vi "E517_InitialisationOfWaveScan.vi"(0 "amplitude":dbl, 5 "FastAxisStart":dbl, 7 "Fast Axis":string="1", 8 "Slow Axis Steps":dbl, 11 "error in":errorcluster, 12 "FastAxisStepsize":dbl, 13 "kineticexposure":dbl) -> (4 "scan time for 1 line/sec":dbl=200.0 format="%.3g", 6 "scan time for 1 area/sec 2":dbl=200.0 format="%.3g", 15 "error out 2":errorcluster)   [LabVIEW 2011]
doc: "This VI initializes and configures the E-710 to perform a XY scan."
uses:
  Utilities/controls/ctlSeqFNs_PI_SysNr.ctl
  Variables/GlobalSetNumberOfDigits_PhysikalInstruments.vi
panel:
  # "E-710 Wavescan Initialization"
  # "This VI initializes and configures the E-710 to perform a XY raster scan. Scan motion in X axis can be uni-\nor bidirectional. Triggerline 1 fires on waveform start."
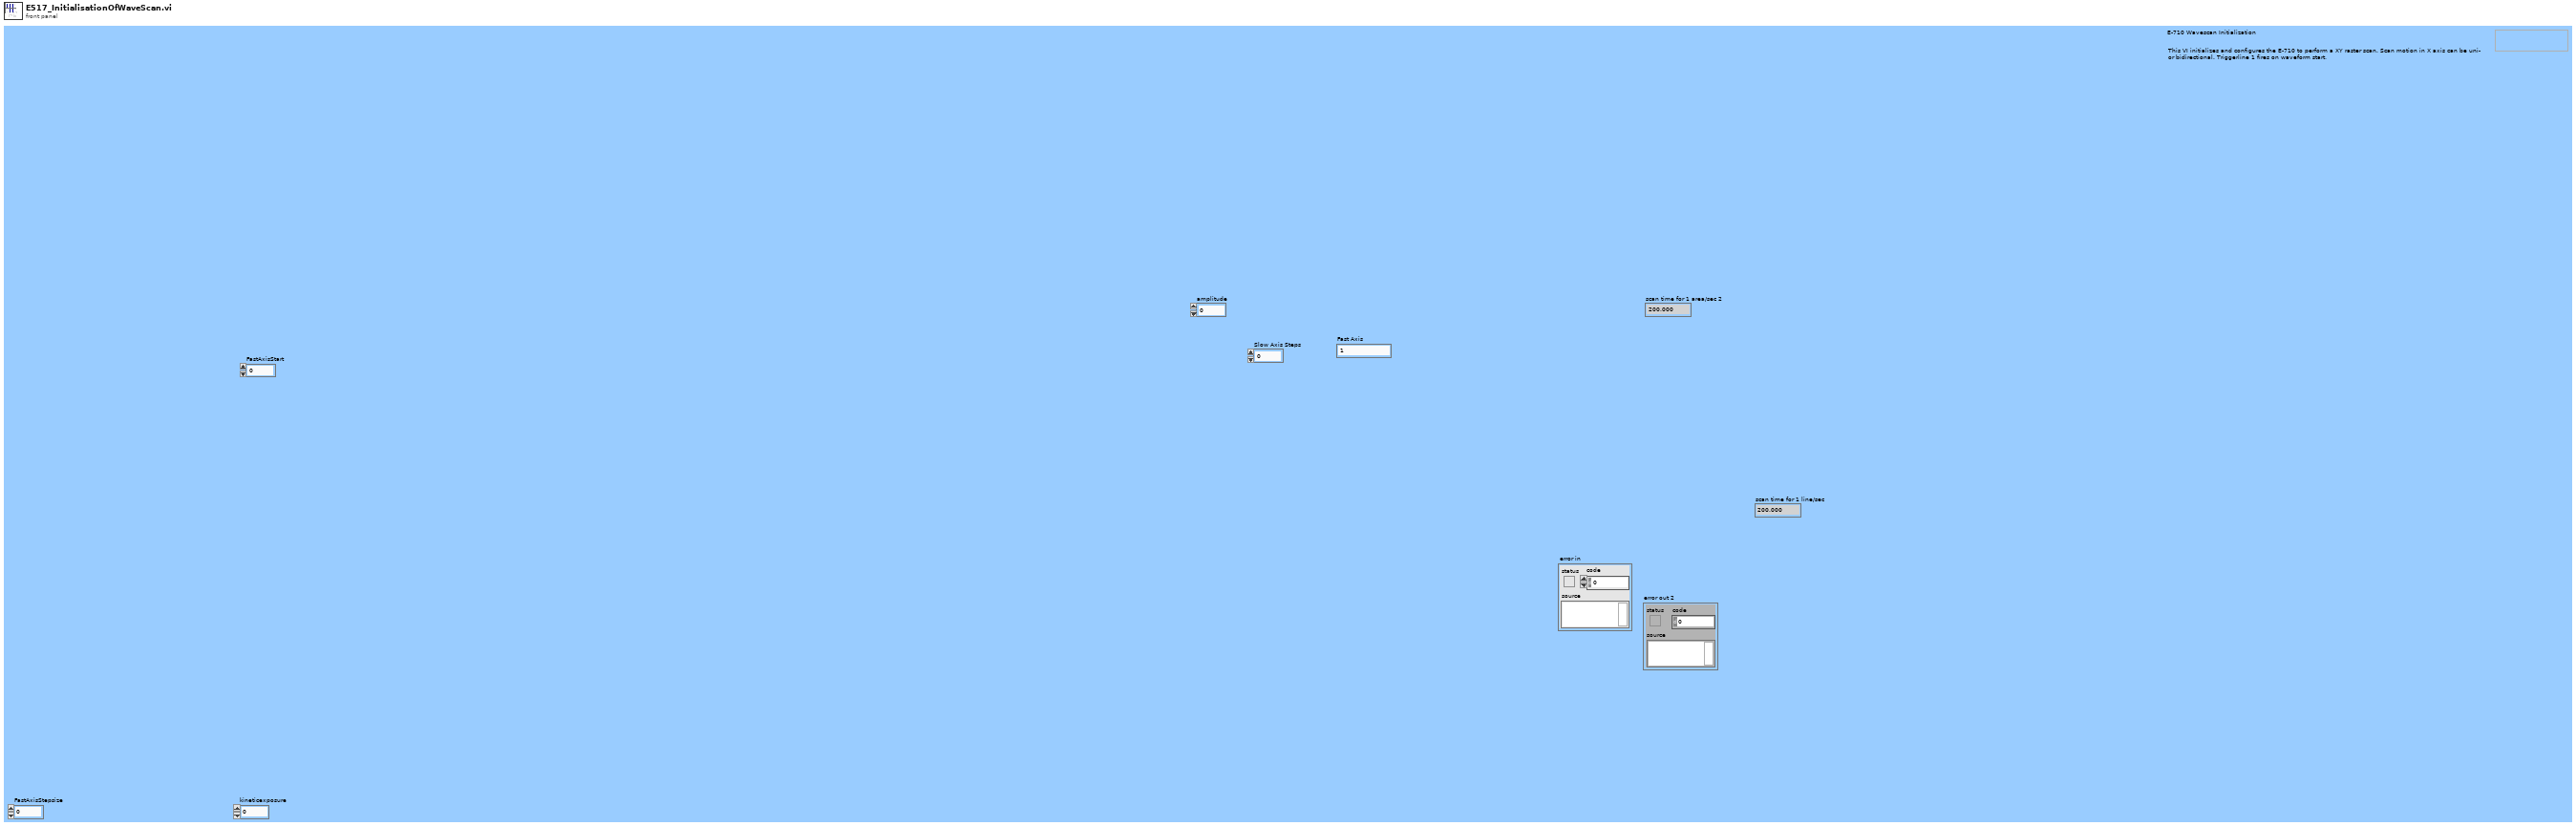
[diagram p1: front panel]
types:
  T1 = enum16{"Exit VI", "Set trigger mode", "Set recordtable rate", "Set wavetable rate", "Write sine", "Read wavetable", "Read recordtable", "Enable/disable wavegen", "Set number of wavegen cycles", "Clear wavetable", "Configure data recorder", "Assign wavetable to wavegen", "Read trigger points", "Set trigger points", "Clear trigger points", "Assign axes to triggerlines", "Write ramp waveform", "Set DDL enable", "Set DDL init", "Set Start at endpoint"}[]
  T2 = typedef "ctlSeqFNs_PI_SysNr.ctl" = enum16{"Zero", "E517", "E710"}
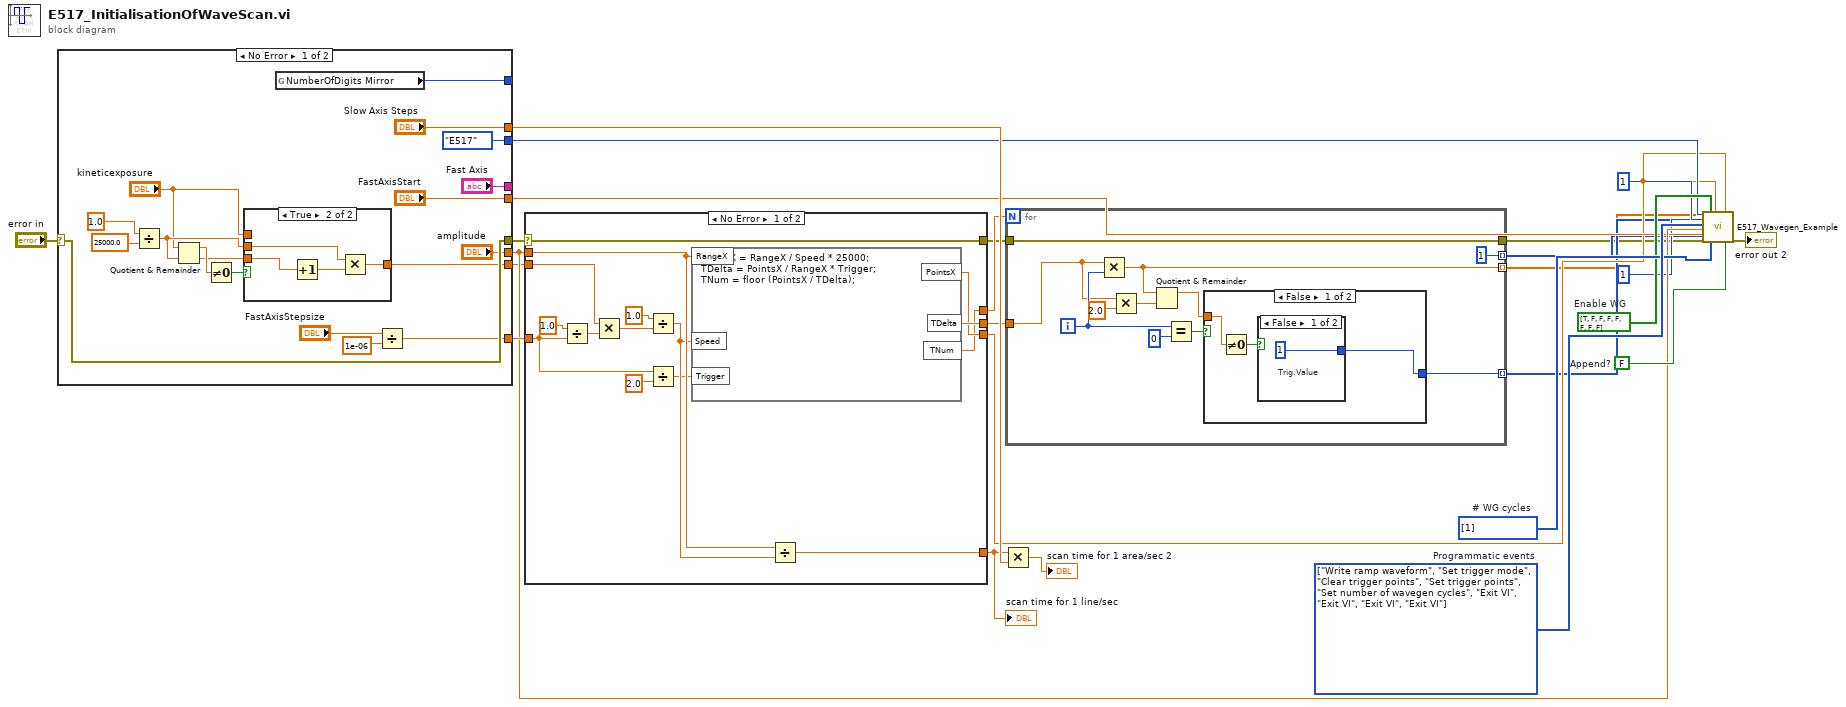
[diagram p0: block diagram]
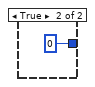
[diagram p2: hidden frame]
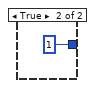
[diagram p3: hidden frame]
diagram:
  w16 = bool[] [TRUE, FALSE, FALSE, FALSE, FALSE, FALSE, FALSE, FALSE]  # Enable WG
  w17 = i32[] [1]  # # WG cycles
  w18 = FALSE  # Append?
  w19 = T1 [enum."Write ramp waveform", enum."Set trigger mode", enum."Clear trigger points", enum."Set trigger points", enum."Set number of wavegen cycles", enum."Exit VI", enum."Exit VI", enum."Exit VI", enum."Exit VI"] items=["Exit VI", "Set trigger mode", "Set recordtable rate", "Set wavetable rate", "Write sine", "Read wavetable", "Read recordtable", "Enable/disable wavegen", "Set number of wavegen cycles", "Clear wavetable", "Configure data recorder", "Assign wavetable to wavegen", "Read trigger points", "Set trigger points", "Clear trigger points", "Assign axes to triggerlines", "Write ramp waveform", "Set DDL enable", "Set DDL init", "Set Start at endpoint"]  # Programmatic events
  n1 = case shown="No Error" "error in" {
    selector: "error in" -> [w39 w49]
    tunnel: ["Fast Axis" _] -> _
    tunnel: [ctlSeqFNs_PI_SysNr."E517" ("STATE") _] -> w15
    tunnel: [w41 _] -> _
    tunnel: ["Slow Axis Steps" _] -> w24
    tunnel: [w39 w49] -> w21
    tunnel: ["amplitude" _] -> w12
    tunnel: [w36 _] -> w22
    tunnel: ["FastAxisStart" _] -> w11
    tunnel: [w27 _] -> w9
    frame No Error {
      n2 = Divide(x=1.0, y=25000.0) -> (x/y=w28:dbl)
      n3 = Quotient & Remainder(x="kineticexposure", y=w28) -> (x-y*floor(x/y)=w31:dbl, floor(x/y)=w29:dbl)
      n4 = Not Equal To 0?(x=w31) -> (x != 0?=w30:bool)
      n5 = case shown="True" w30 {
        tunnel: w29 -> [_ w48]
        tunnel: w28 -> [_ w46]
        tunnel: [w44 w45] -> w27
        tunnel: "kineticexposure" -> [w44 _]
        frame False {
        }
        frame True {
          n6 = Increment(x=w48) -> (x+1=w47:dbl)
          n7 = Multiply(x=w46, y=w47) -> (x*y=w45:dbl)
        }
      }
      n8 = global read "GlobalSetNumberOfDigits_PhysikalInstruments.vi" "NumberOfDigits Mirror"() -> (w41:i32)
      n9 = Divide(x="FastAxisStepsize", y=1e-06) -> (x/y=w36:dbl)
    }
    frame Error {
    }
  }
  n10 = case shown="No Error" w21 {
    selector: w21 -> [w62 _]
    tunnel: [w64 _] -> w6
    tunnel: w12 -> [w56 _]
    tunnel: w22 -> [w53 _]
    tunnel: [w63 _] -> w8
    tunnel: [w62 _] -> w5
    tunnel: [w61 _] -> w20
    tunnel: w9 -> [w54 _]
    tunnel: [w50 _] -> w7
    frame No Error {
      n11 = Divide(x=1.0, y=w53) -> (x/y=w59:dbl)
      n12 = Multiply(x=w54, y=w59) -> (x*y=w58:dbl)
      n13 = Divide(x=1.0, y=w58) -> (x/y=w55:dbl)
      n14 = Divide(x=w53, y=2.0) -> (x/y=w51:dbl)
      n15 = formula code="PointsX = RangeX / Speed * 25000;\nTDelta = PointsX / RangeX * Trigger;\nTNum = floor (PointsX / TDelta);"("RangeX"=w56, "Speed"=w55, "Trigger"=w51) -> ("PointsX"=w63:dbl, "TDelta"=w64:dbl, "TNum"=w50:dbl)
      n16 = Divide(x=w56, y=w55) -> (x/y=w61:dbl)
    }
    frame Error {
    }
  }
  "scan time for 1 line/sec" <- w20
  n17 = Multiply(x=w20, y=w24) -> (x*y=→"scan time for 1 area/sec 2":dbl)
  n18 = for {
    N: w7 -> [_]
    tunnel: w6 -> [w66]
    tunnel: [w69] -> w3 mode=indexing
    tunnel: [w75] -> w4 mode=indexing
    tunnel: w5 -> [w70]
    tunnel: [w70] -> w1
    tunnel: [1] -> w2 mode=indexing
    i -> [w73]
    n19 = Multiply(x=w66, y=w73) -> (x*y=w69:dbl)
    n20 = Multiply(x=w66, y=2.0) -> (x*y=w68:dbl)
    n21 = Quotient & Remainder(x=w69, y=w68) -> (x-y*floor(x/y)=w74:dbl)  [unwired: 1 out]
    n22 = Equal?(x=w73, y=0) -> (x = y?=w71:bool)
    n23 = case shown="False" w71 {
      tunnel: [w78 1] -> w75
      tunnel: w74 -> [w77 _]
      frame False {
        n24 = Not Equal To 0?(x=w77) -> (x != 0?=w76:bool)
        n25 = case shown="False" w76 {
          tunnel: [1 0] -> w78
          frame False {
            # "Trig.Value"
          }
          frame True {
          }
        }
      }
      frame True {
      }
    }
  }
  n26 = call "E517_Wavegen_Example.vi"("System no."=w15, "# Wavegenerators"=1, "Programmatic events"=w19, 3:w12, 4:w11, "error in"=w1, "Enabled"=w16, "# WG cycles"=w17, 8:w8, 10:1 ("Xo"), "Firing Wavepoints"=w2, 12:w8, "Append?"=w18, 14:w3, 15:w4) -> ("Error out"=→"error out 2":errorcluster)  [unwired: 1 in, 3 out]
